vi "Enums.vi"() -> ()   [LabVIEW 2020]
panel:
  out "Modern Enum Indicator":T1(ring)
  out "NXG Enum Indicator":T1(ring)
  out "Silver Enum Indicator":T1(ring)
  out "System Enum Indicator":T1(ring)
  out "Classic Enum Indicator":T1(ring)
  in  "Classic Enum":T1(ring)
  in  "System Enum":T1(ring)
  in  "Silver Enum":T1(ring)
  in  "NXG Enum":T1(ring)
  in  "Modern Enum":T1(ring)
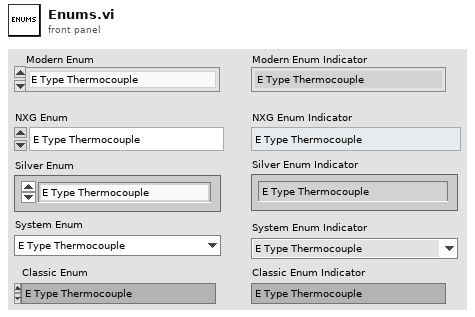
[diagram p1: front panel]
types:
  T1 = enum16{"E Type Thermocouple", "J Type Thermocouple", "K Type Thermocouple", "N Type Thermocouple", "R Type Thermocouple", "S Type Thermocouple", "T Type Thermocouple", "B Type Thermocouple"}
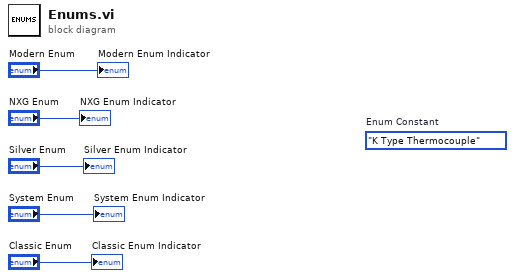
[diagram p0: block diagram]
diagram:
  (unwired) T1."K Type Thermocouple"  # Enum Constant
  "Classic Enum Indicator" <- "Classic Enum"
  "System Enum Indicator" <- "System Enum"
  "Silver Enum Indicator" <- "Silver Enum"
  "NXG Enum Indicator" <- "NXG Enum"
  "Modern Enum Indicator" <- "Modern Enum"
